vi "Set Identifier.vi"(10 "Identifier":string, 11 "Reply Protocol Base in":refnum<class "Reply Protocol Base.lvclass">) -> (3 "Reply Protocol Base out":refnum<class "Reply Protocol Base.lvclass">)   [LabVIEW 2023, in "HAL GOOP4.lvlib" / "Reply Protocol Base.lvclass"]
uses:
  Reply Protocol Base.lvclass
  Reply Protocol Base.lvclass/Reply Protocol Base.ctl
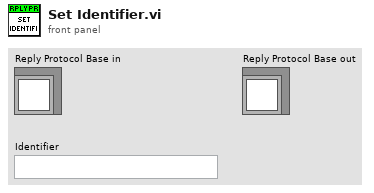
[diagram p1: front panel]
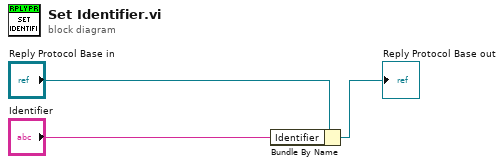
[diagram p0: block diagram]
diagram:
  n1 = Bundle By Name(cluster="Reply Protocol Base in", "Identifier"="Identifier") -> (→"Reply Protocol Base out":refnum<class "Reply Protocol Base.lvclass">)
